vi "Get BlackLevelRange.vi"(8 "error in (no error)":errorcluster, 11 "TLCamera reference in":refnum<k24>) -> (0 "error out":errorcluster, 1 "Maximum":u32, 2 "Minimum":u32, 3 "TLCamera reference out":refnum<k24>)   [LabVIEW 2022 SP3]
uses:
  I:/.shortcut-targets-by-id/1riZacJd_1_jmKfGgrjDuP7KcecvMS3i2/Xiao research group/Programs/XYZRecorrection/Scientific Camera Interfaces/SDK/DotNet Toolkit/dlls/Managed_64_lib/Thorlabs.TSI.TLCamera.dll
  SDK/DotNet Toolkit/dlls/Managed_64_lib/Thorlabs.TSI.TLCamera.dll
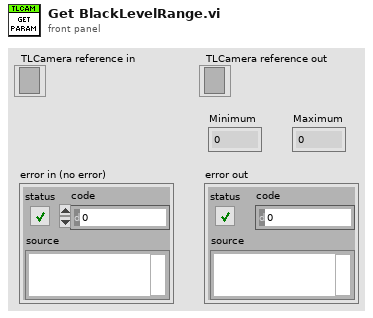
[diagram p1: front panel]
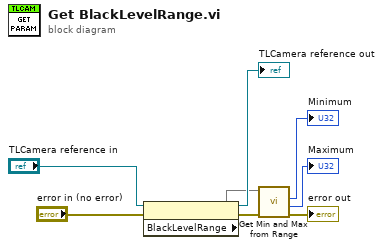
[diagram p0: block diagram]
diagram:
  n1 = property(reference="TLCamera reference in", error in="error in (no error)") -> (reference out=→"TLCamera reference out":refnum<k24>, error out=w4:errorcluster, "BlackLevelRange"=w5)
  n2 = call "Get Min and Max from Range.vi"("error in (no error)"=w4, "Thorlabs.TSI.CoreInterfaces.Range`1[[System.UInt32, mscorlib, Version=4.0.0.0, Culture=neutral, PublicKeyToken=b77a5c561934e089]]"=w5) -> ("error out"=→"error out":errorcluster, "Maximum"=→"Maximum":u32, "Minimum"=→"Minimum":u32)  [unwired: 7 in]
